vi "Acquire.vi"(8 "error in (no error)":errorcluster, 10 "Acquire":bool, 11 "Top Level in":refnum<class "Top Level.lvclass">) -> (0 "error out":errorcluster, 3 "Top Level out":refnum<class "Top Level.lvclass">)   [LabVIEW 2021, in "Top Level.lvlib" / "Top Level.lvclass"]
uses:
  Top Level.lvclass
  Top Level.lvclass/Top Level.ctl
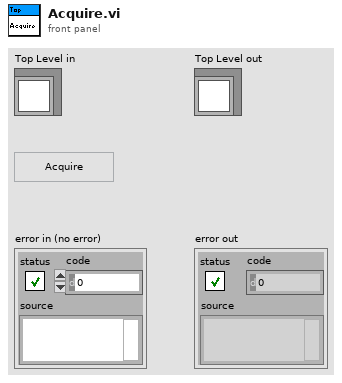
[diagram p1: front panel]
types:
  T1 = enum8{"Enabled", "Disabled", "Disabled and Grayed Out"}
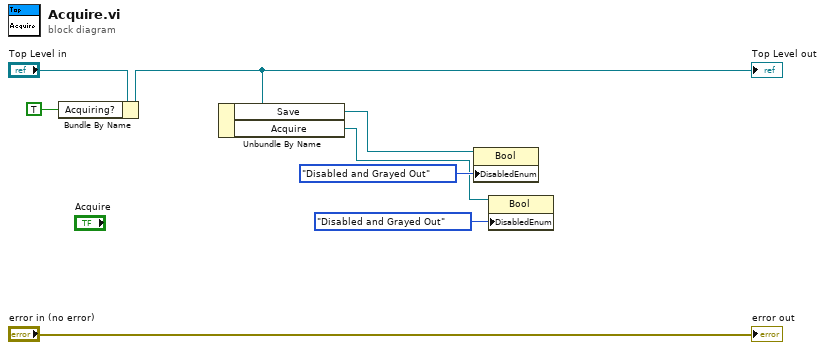
[diagram p0: block diagram]
diagram:
  n1 = Bundle By Name(cluster="Top Level in", "Acquiring?"=TRUE) -> (w5:refnum<class "Top Level.lvclass">)
  "Top Level out" <- w5
  n2 = Unbundle By Name(w5) -> ("Save"=w4:refnum<vi>, "Acquire"=w1:refnum<vi>)
  n3 = property class="Bool"(reference=w4, "DisabledEnum"=T1."Disabled and Grayed Out" ("Disabled")) -> ()  [unwired: 1 in, 2 out]
  n4 = property class="Bool"(reference=w1, "DisabledEnum"=T1."Disabled and Grayed Out" ("Disabled")) -> ()  [unwired: 1 in, 2 out]
  "error out" <- "error in (no error)"
